vi "Set Order Handler.vi"(8 "error in (no error)":errorcluster, 10 "Order Handler":refnum<class "Job Handler.lvclass">, 11 "Customer In":refnum<class "Customer.lvclass">) -> (0 "error out":errorcluster, 3 "Customer Out":refnum<class "Customer.lvclass">)   [LabVIEW 2020, in "Customer.lvclass"]
uses:
  Customer.lvclass
  C:/Program Files (x86)/National Instruments/LabVIEW 2020/vi.lib/Astemes/Triarc Framework/Process/Process.lvclass
  Process Job/Job Handler.lvclass
  <vilib>/Astemes/Triarc Framework/Process/Process.lvclass/Process.ctl
  Customer.lvclass/Customer.ctl
  <vilib>/Astemes/Triarc Framework/Process/Private/SubVIs/Handle Debug Data.vi
  <vilib>/Astemes/Triarc Framework/Logging/Log Debug.vi
  <vilib>/AdvancedString/1D String Array to Delimited String.vi
  <vilib>/Utility/High Resolution Relative Seconds.vi
  <vilib>/Astemes/Triarc Framework/Process/Public/Read Name.vi
  <vilib>/Astemes/Triarc Framework/Callback/Callback.lvclass
  <vilib>/Astemes/Triarc Framework/Process/Process.lvclass
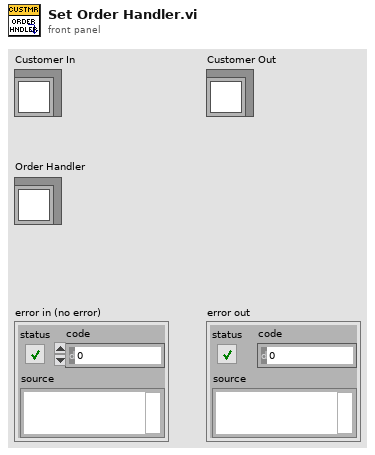
[diagram p1: front panel]
types:
  T1 = typedef "TF.lvlib/Process.lvclass/API Mode.ctl" = enum16{"Send Message", "Handle Message"}
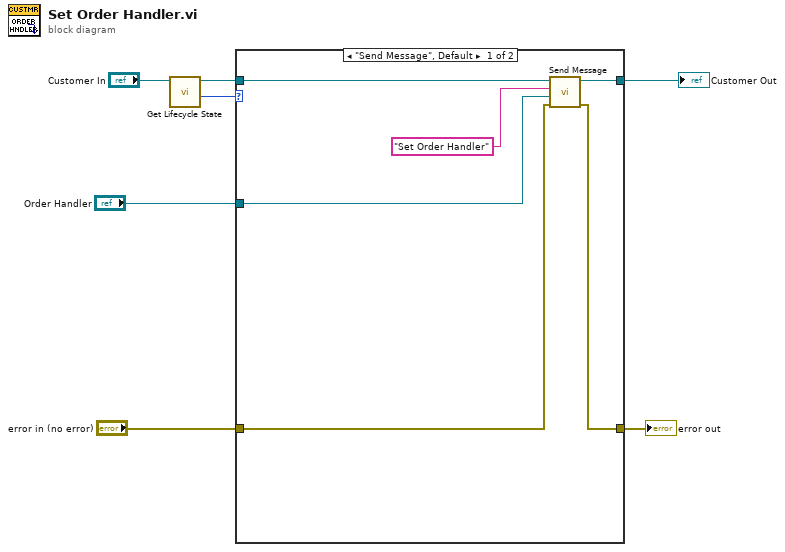
[diagram p0: block diagram]
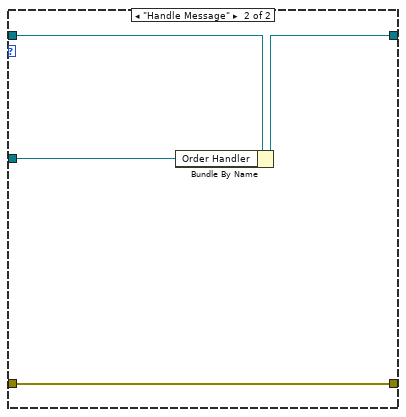
[diagram p2: hidden frame]
diagram:
  n1 = call <vilib>:"Get Lifecycle State.vi"("Process In"="Customer In") -> ("API Mode"=w3:T1, "Process Out"=w6:refnum<class "Customer.lvclass">)  [unwired: 7 in, 2 out]
  n2 = case shown="\"Send Message\", Default" w3 {
    tunnel: w6 -> [w13 w17]
    tunnel: [w12 w15] -> w5
    tunnel: "error in (no error)" -> [w8 w16]
    tunnel: [w9 w16] -> w4
    tunnel: "Order Handler" -> [w11 w14]
    frame "Send Message", Default {
      n3 = call <vilib>:"Send Message.vi"("error in (no error)"=w8, "Message Data"=w11, "Message"="Set Order Handler" ("API Message"), "Process In"=w13) -> ("error out"=w9:errorcluster, "Process Out"=w12:refnum<class "Customer.lvclass">)  [unwired: 6 in]
    }
    frame "Handle Message" {
      n4 = Bundle By Name(cluster=w17, "Order Handler"=w14) -> (w15:refnum<class "Customer.lvclass">)
    }
  }
  "error out" <- w4
  "Customer Out" <- w5
